vi "Create Hyperlink.vi"(0 "Work Sheet":refnum<k7>, 1 "File Path":path, 5 "Sheet Name":string, 7 "Link Cell 1":string, 9 "Link Cell 2":string, 11 "error in":errorcluster) -> (15 "error out":errorcluster)   [LabVIEW 2017]
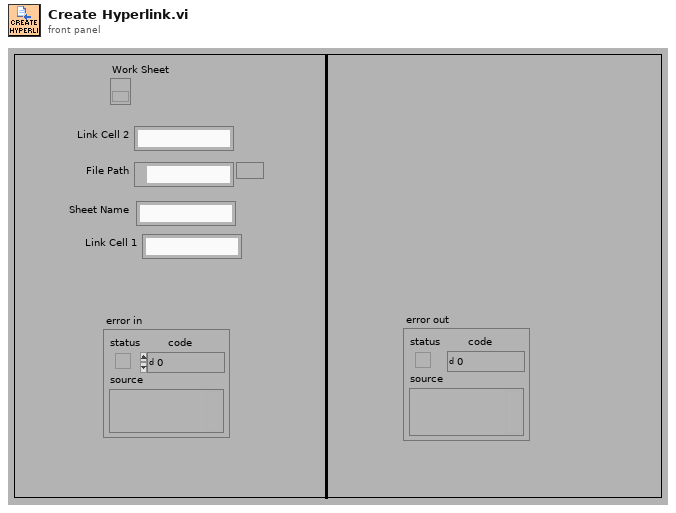
[diagram p1: front panel]
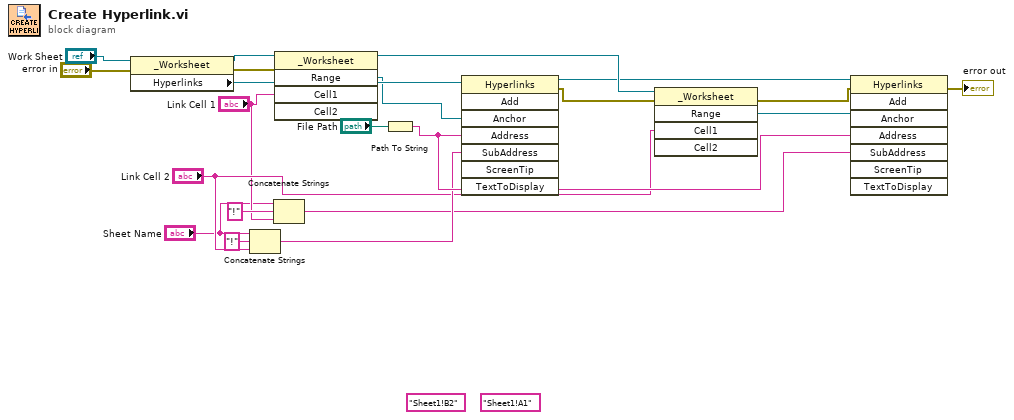
[diagram p0: block diagram]
diagram:
  (unwired) "Sheet1!A1"
  (unwired) "Sheet1!B2"
  n1 = property class="_Worksheet"(reference="Work Sheet", error in="error in") -> (reference out=w21:refnum<k7>, error out=w20:errorcluster, "Hyperlinks"=w19:refnum<k7>)
  n2 = Concatenate Strings("Sheet Name", "!" ("string"), "Link Cell 2") -> (w7:string)
  n3 = Concatenate Strings("Sheet Name", "!" ("string"), "Link Cell 1") -> (w3:string)
  n4 = invoke class="_Worksheet" method="Range"(reference=w21, error in=w20, "Cell1"="Link Cell 1") -> (reference out=w17:refnum<k7>, "Range"=w18:refnum<k7>)  [unwired: 2 in, 3 out]
  n5 = Path To String(path="File Path") -> (string=w13:string)
  n6 = invoke class="Hyperlinks" method="Add"(reference=w19, "Anchor"=w18, "Address"=w13, "SubAddress"=w7) -> (reference out=w14:refnum<k7>, error out=w16:errorcluster)  [unwired: 4 in, 6 out]
  n7 = invoke class="_Worksheet" method="Range"(reference=w17, error in=w16, "Cell1"="Link Cell 2") -> (error out=w2:errorcluster, "Range"=w15:refnum<k7>)  [unwired: 2 in, 3 out]
  n8 = invoke class="Hyperlinks" method="Add"(reference=w14, error in=w2, "Anchor"=w15, "Address"=w13, "SubAddress"=w3) -> (error out=→"error out":errorcluster)  [unwired: 3 in, 7 out]
